vi "XYcordenadas_a_string_float.vi"(8 "fin de cadena":string=" S", 9 "decimales":i16, 10 "y":dbl, 11 "x":dbl) -> (2 "String":string, 5 "ok":bool)   [LabVIEW 2017]
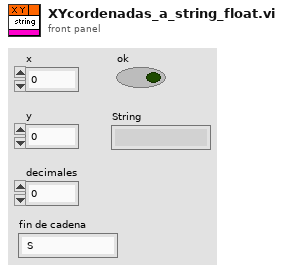
[diagram p1: front panel]
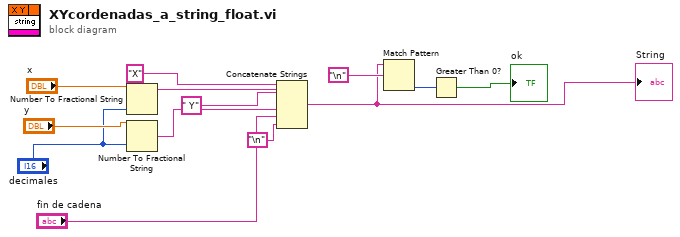
[diagram p0: block diagram]
diagram:
  n1 = Number To Fractional String(number="x", precision (6)="decimales") -> (F-format string=w5:string)  [unwired: 2 in]
  n2 = Number To Fractional String(number="y", precision (6)="decimales") -> (F-format string=w7:string)  [unwired: 2 in]
  n3 = Concatenate Strings("X" ("string"), w5, " Y" ("string"), w7, "fin de cadena", "\n") -> (w10:string)
  "String" <- w10
  n4 = Match Pattern(string=w10, regular expression="\n") -> (offset past match=w12:i32)  [unwired: 1 in, 3 out]
  n5 = Greater Than 0?(x=w12) -> (x > 0?=→"ok":bool)
